vi "group_data.vi"(1 "VISA Resource Names":refnum<visa-resource-name>[](array[refnum]), 2 "Input Values":dbl[](array[numeric])) -> (0 "Grouped Data":T1(array[cluster]))   [LabVIEW 2019]
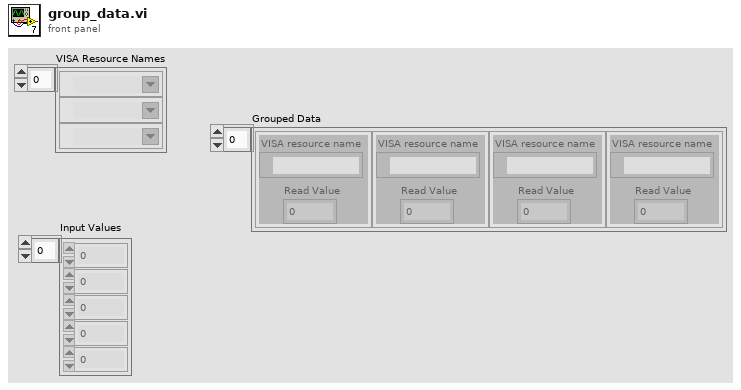
[diagram p1: front panel]
types:
  T1 = cluster{"Read Value":dbl, "VISA resource name":refnum<visa-resource-name>}[]
  T2 = cluster{"Numeric":dbl, "VISA resource name":refnum<visa-resource-name>}
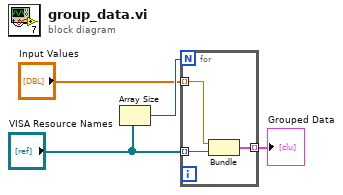
[diagram p0: block diagram]
diagram:
  n1 = Array Size(array="VISA Resource Names") -> (size(s)=w3:i32)
  n2 = for {
    N: w3 -> [_]
    tunnel: "VISA Resource Names" -> [w7] mode=indexing
    tunnel: [w6] -> w1 mode=indexing
    tunnel: "Input Values" -> [w5] mode=indexing
    n3 = Bundle("Numeric"=w5, "VISA resource name"=w7) -> (w6:T2)  [unwired: 1 in]
  }
  "Grouped Data" <- w1
